vi "ma_concatenate waveforms (dual).vi"(0 "Waveform A0 in":waveform(dbl)={"t0"=timestamp(0 s since 1904-01-01), "dt"=0.0, "Y"=[]}, 5 "Waveform B0 in":waveform(dbl)={"t0"=timestamp(0 s since 1904-01-01), "dt"=0.0, "Y"=[]}, 7 "Waveform A1 in":waveform(dbl)={"t0"=timestamp(0 s since 1904-01-01), "dt"=0.0, "Y"=[]}, 9 "Waveform B1 in":waveform(dbl)={"t0"=timestamp(0 s since 1904-01-01), "dt"=0.0, "Y"=[]}, 11 "error in":errorcluster) -> (4 "Waveform A out":waveform(dbl), 6 "Waveform B out":waveform(dbl), 15 "error out":errorcluster)   [LabVIEW 2020, in "NI_MAPro.lvlib"]
uses:
  NI_MAPro.lvlib
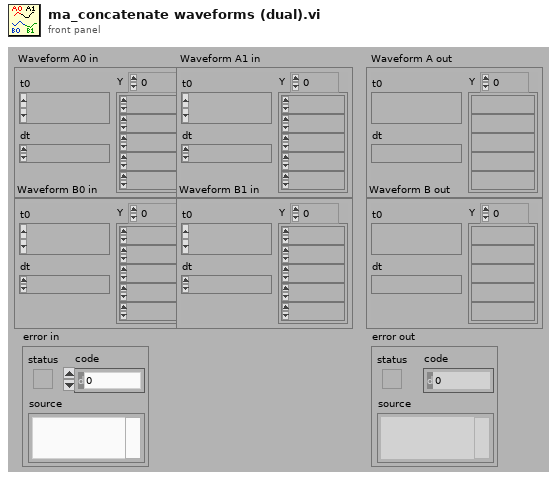
[diagram p1: front panel]
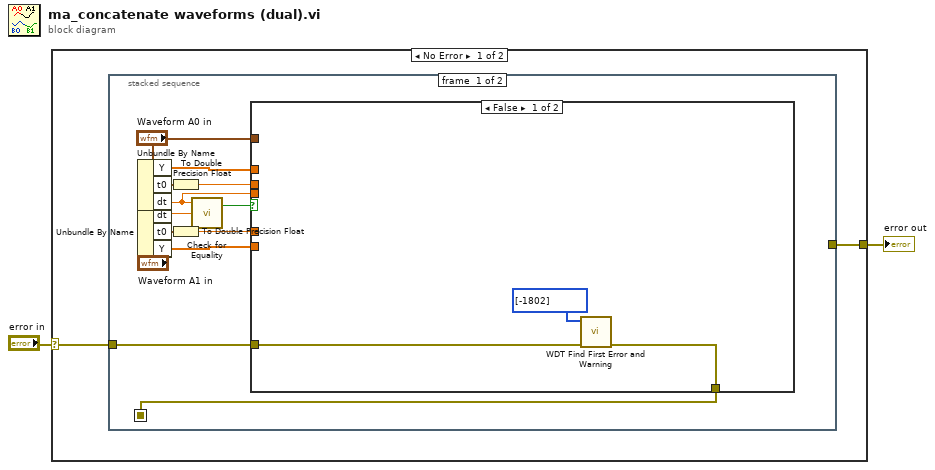
[diagram p0: block diagram]
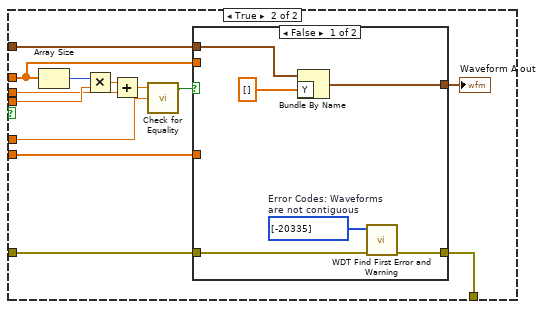
[diagram p2: hidden frame]
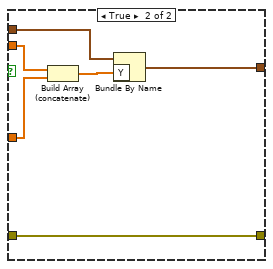
[diagram p3: hidden frame]
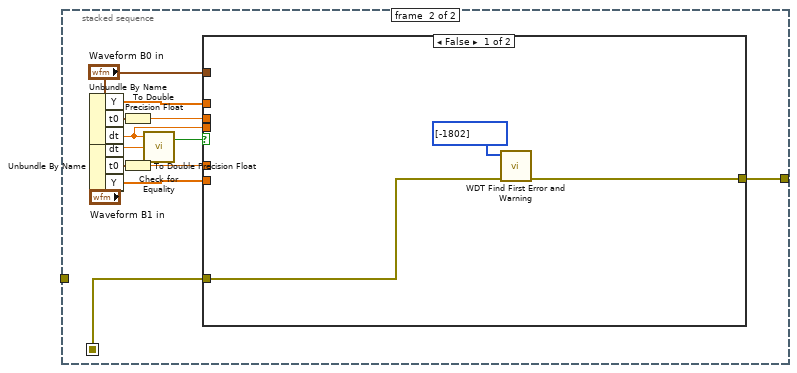
[diagram p4: hidden frame]
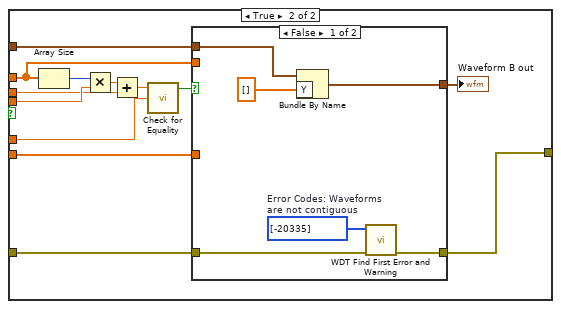
[diagram p5: hidden frame]
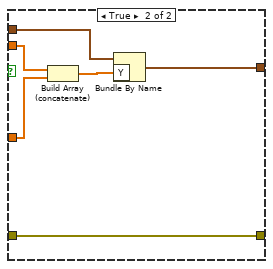
[diagram p6: hidden frame]
diagram:
  n1 = case shown="No Error" "error in" {
    selector: "error in" -> [w4 w87]
    tunnel: [w3 w87] -> w1
    frame No Error {
      n2 = stacked-sequence {
        seq-local: [w7 _] -> [_ w51]
        tunnel: w4 -> [w15 _]
        tunnel: [_ w50] -> w3
        frame #0 {
          n3 = Unbundle By Name("Waveform A0 in") -> ("Y"=w13:dbl[], "t0"=w5:timestamp, "dt"=w12:dbl)
          n4 = Unbundle By Name("Waveform A1 in") -> ("dt"=w17:dbl, "t0"=w6:timestamp, "Y"=w9:dbl[])
          n5 = To Double Precision Float(number=w5) -> (double precision float=w11:dbl)
          n6 = To Double Precision Float(number=w6) -> (double precision float=w10:dbl)
          n7 = call "Check for Equality.vi"("n2"=w17, "n1"=w12) -> ("equal?"=w14:bool)  [unwired: 1 in, 1 out]
          n8 = case shown="False" w14 {
            tunnel: w15 -> [w20 w24]
            tunnel: w13 -> [_ w26]
            tunnel: w12 -> [_ w32]
            tunnel: w11 -> [_ w30]
            tunnel: w10 -> [_ w28]
            tunnel: w9 -> [_ w25]
            tunnel: "Waveform A0 in" -> [_ w27]
            tunnel: [w18 w23] -> w7
            frame False {
              n9 = call "WDT Find First Error and Warning.vi"("error in (no error)"=w20, "Error Codes"=i32[] [-1802]) -> ("error out"=w18:errorcluster)  [unwired: 4 in, 1 out]
            }
            frame True {
              n10 = Array Size(array=w26) -> (size(s)=w33:i32)
              n11 = Multiply(x=w33, y=w32) -> (x*y=w31:dbl)
              n12 = Add(x=w31, y=w30) -> (x+y=w29:dbl)
              n13 = call "Check for Equality.vi"("n2"=w28, "n1"=w29) -> ("equal?"=w21:bool)  [unwired: 1 in, 1 out]
              n14 = case shown="False" w21 {
                tunnel: w26 -> [_ w45]
                tunnel: w25 -> [_ w44]
                tunnel: w27 -> [w38 w42]
                tunnel: [w37 w41] -> w22
                tunnel: [w36 w40] -> w23
                tunnel: w24 -> [w34 w40]
                frame False {
                  w35 = i32[] [-20335]  # Error Codes: Waveforms are not contiguous
                  n15 = Bundle By Name(cluster=w38, "Y"=dbl[] []) -> (w37:waveform(dbl))
                  n16 = call "WDT Find First Error and Warning.vi"("error in (no error)"=w34, "Error Codes"=w35) -> ("error out"=w36:errorcluster)  [unwired: 4 in, 1 out]
                }
                frame True {
                  n17 = Build Array (concatenate)(w45, w44) -> (w43:dbl[])
                  n18 = Bundle By Name(cluster=w42, "Y"=w43) -> (w41:waveform(dbl))
                }
              }
              "Waveform A out" <- w22
            }
          }
        }
        frame #1 {
          n19 = Unbundle By Name("Waveform B0 in") -> ("Y"=w56:dbl[], "t0"=w46:timestamp, "dt"=w55:dbl)
          n20 = Unbundle By Name("Waveform B1 in") -> ("dt"=w58:dbl, "t0"=w47:timestamp, "Y"=w52:dbl[])
          n21 = To Double Precision Float(number=w46) -> (double precision float=w54:dbl)
          n22 = To Double Precision Float(number=w47) -> (double precision float=w53:dbl)
          n23 = call "Check for Equality.vi"("n2"=w58, "n1"=w55) -> ("equal?"=w57:bool)  [unwired: 1 in, 1 out]
          n24 = case shown="False" w57 {
            tunnel: w51 -> [w60 w64]
            tunnel: w56 -> [_ w67]
            tunnel: w55 -> [_ w73]
            tunnel: w54 -> [_ w71]
            tunnel: w53 -> [_ w69]
            tunnel: w52 -> [_ w66]
            tunnel: "Waveform B0 in" -> [_ w65]
            tunnel: [w59 w63] -> w50
            frame False {
              n25 = call "WDT Find First Error and Warning.vi"("error in (no error)"=w60, "Error Codes"=i32[] [-1802]) -> ("error out"=w59:errorcluster)  [unwired: 4 in, 1 out]
            }
            frame True {
              n26 = Array Size(array=w67) -> (size(s)=w74:i32)
              n27 = Multiply(x=w74, y=w73) -> (x*y=w72:dbl)
              n28 = Add(x=w72, y=w71) -> (x+y=w70:dbl)
              n29 = call "Check for Equality.vi"("n2"=w69, "n1"=w70) -> ("equal?"=w68:bool)  [unwired: 1 in, 1 out]
              n30 = case shown="False" w68 {
                tunnel: w67 -> [_ w86]
                tunnel: w66 -> [_ w85]
                tunnel: w65 -> [w79 w83]
                tunnel: [w78 w82] -> w62
                tunnel: [w77 w81] -> w63
                tunnel: w64 -> [w75 w81]
                frame False {
                  w76 = i32[] [-20335]  # Error Codes: Waveforms are not contiguous
                  n31 = Bundle By Name(cluster=w79, "Y"=dbl[] []) -> (w78:waveform(dbl))
                  n32 = call "WDT Find First Error and Warning.vi"("error in (no error)"=w75, "Error Codes"=w76) -> ("error out"=w77:errorcluster)  [unwired: 4 in, 1 out]
                }
                frame True {
                  n33 = Build Array (concatenate)(w86, w85) -> (w84:dbl[])
                  n34 = Bundle By Name(cluster=w83, "Y"=w84) -> (w82:waveform(dbl))
                }
              }
              "Waveform B out" <- w62
            }
          }
        }
      }
    }
    frame Error {
    }
  }
  "error out" <- w1
